vi "save.vi"(4 "additional vol. [ml]":dbl=11.0, 6 "pipette vol. [ml]":dbl=0.2148, 7 "CA-Name":string, 8 "calibration vol. [ml]":dbl=10670.0, 9 "humidity [%]":dbl, 10 "pressure [mbar]":dbl, 11 "temperature [°C]":dbl) -> ()   [LabVIEW 2013]
uses:
  Instance           1 12Saved   save .vi
  <vilib>/Utility/config.llb/Write Key (Double).vi
  <vilib>/Utility/config.llb/NI_LVConfig.lvlib
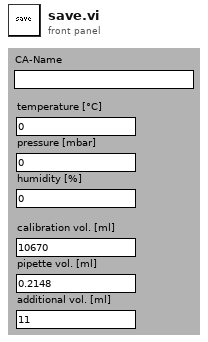
[diagram p1: front panel]
types:
  T1 = typedef "NI_LVConfig.lvlib/Config Data RefNum.ctl" = refnum<k1>
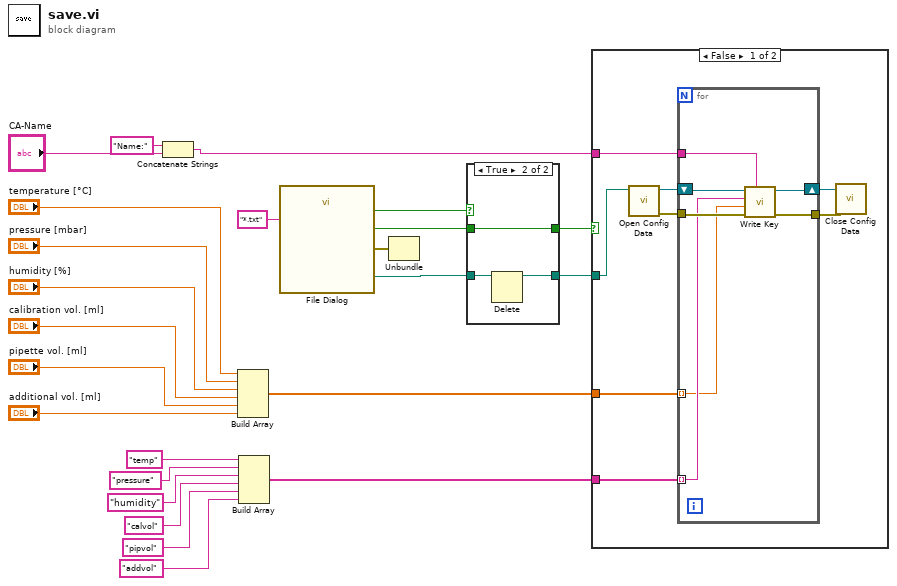
[diagram p0: block diagram]
diagram:
  n1 = Concatenate Strings("Name:" ("string"), "CA-Name") -> (w7:string)
  n2 = Build Array("temperature [°C]", "pressure [mbar]", "humidity [%]", "calibration vol. [ml]", "pipette vol. [ml]", "additional vol. [ml]") -> (w12:dbl[])
  n3 = Build Array("temp", "pressure", "humidity", "calvol", "pipvol", "addvol") -> (w11:string[])
  n4 = call "File Dialog"("pattern (all files)"="*.txt") -> ("selected path"=w6:path, "exists"=w5:bool, "cancelled"=w4:bool, "error out"=w1:errorcluster)  [unwired: 11 in]
  n5 = Unbundle(w1) -> ()  [unwired: 3 out]
  n6 = case shown="True" w5 {
    tunnel: w6 -> [w25 w29]
    tunnel: w4 -> [w26 w27]
    tunnel: [w25 w28] -> w3
    tunnel: [w26 w27] -> w2
    frame False {
    }
    frame True {
      n7 = Delete(path (use dialog)=w29) -> (deleted path=w28:path)  [unwired: 4 in, 2 out]
    }
  }
  n8 = case shown="False" w2 {
    tunnel: w12 -> [w35 _]
    tunnel: w11 -> [w34 _]
    tunnel: w7 -> [w33 _]
    tunnel: w3 -> [w30 _]
    frame False {
      n9 = call <vilib>:"Open Config Data.vi"("configuration file path"=w30) -> ("error out"=w36:errorcluster, "refnum"=w37:T1)  [unwired: 8 in, 1 out]
      n10 = for {
        tunnel: w36 -> [w42]
        shift-right: [w43] -> w32
        shift-left: w37 -> [w44]
        tunnel: [w41] -> w31
        tunnel: w35 -> [w39] mode=indexing
        tunnel: w34 -> [w40] mode=indexing
        tunnel: w33 -> [w38]
        n11 = call-poly <vilib>:"Write Key.vi"("section"=w38, "error in (no error)"=w42, "value"=w39, "key"=w40, "refnum"=w44) -> ("error out"=w41:errorcluster, "refnum out"=w43:T1)  [unwired: 4 in, 1 out]
      }
      n12 = call <vilib>:"Close Config Data.vi"("error in (no error)"=w31, "refnum"=w32) -> ()  [unwired: 8 in, 2 out]
    }
    frame True {
    }
  }
